vi "Connect.vi"(8 "Error In":errorcluster, 11 "Arduino Port":refnum<visa-resource-name>) -> (0 "Error Out":errorcluster, 3 "Arduino Port out":refnum<visa-resource-name>)   [LabVIEW 2016]
uses:
  <vilib>/Instr/_visa.llb/VISA Configure Serial Port (Instr).vi
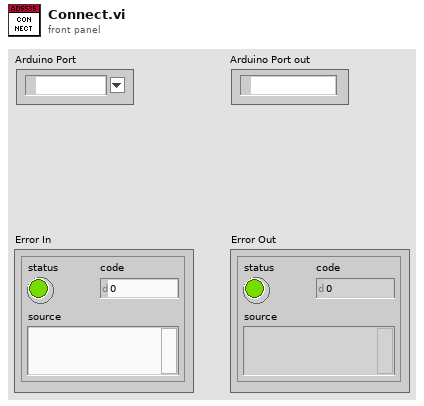
[diagram p1: front panel]
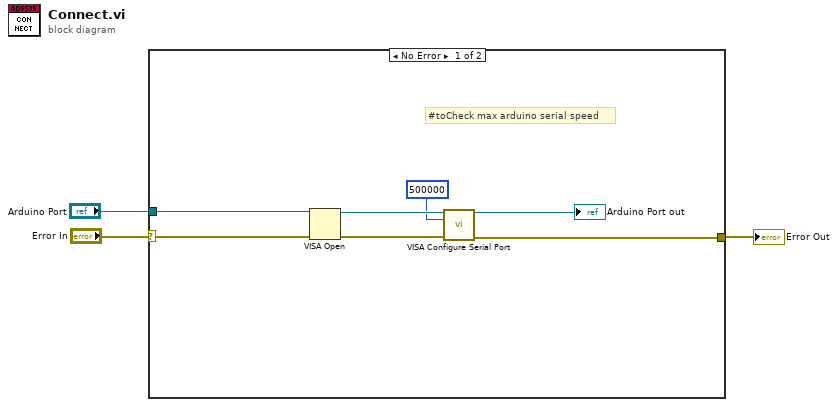
[diagram p0: block diagram]
diagram:
  n1 = case shown="No Error" "Error In" {
    selector: "Error In" -> [w8 w11]
    tunnel: [w7 w11] -> w2
    tunnel: "Arduino Port" -> [w6 _]
    frame No Error {
      # "#toCheck max arduino serial speed"
      n2 = VISA Open(error in (no error)=w8, VISA resource name=w6) -> (VISA resource name=w10:refnum<visa-resource-name>, error out=w9:errorcluster)  [unwired: 3 in]
      n3 = call-poly "VISA Configure Serial Port"("VISA resource name"=w10, "baud rate (9600)"=u32 500000, "error in (no error)"=w9) -> ("VISA resource name out"=→"Arduino Port out":refnum<visa-resource-name>, "error out"=w7:errorcluster)  [unwired: 11 in]
    }
    frame Error {
    }
  }
  "Error Out" <- w2
